vi "BLED1112-Rx Packet parser (RESPONSE-GAP).vi"(5 "message package":u8[](array[numeric])=[0, 3, 6, 3, 0, 0, 0] format="%02x") -> (0 "message out":u8[](array[numeric])=[0, 3, 6, 3, 0, 0, 0] format="%02x", 1 "Packet OK":bool, 2 "Data Structure":T1={"Message Type (Response)"=0, "Payload length"=3, "Message class"=6, "Message ID"=3, "result"=0, "connection_handle"=0} {"Message class" format="%02x"; "connection_handle" format="%02x"; "result" format="%04x"; "Message ID" format="%02x"; "Message Type (Response)" format="%02x" items=["Command / Response"=0, "Event"=128]})   [LabVIEW 2015]
uses:
  Control-BLED Rx (RESPONSE-GAP).ctl
  Lib_Bled112 toolkit/type_def/message_type.ctl
panel:
  # "Rx Packet parser (RESPONSE GAP)"
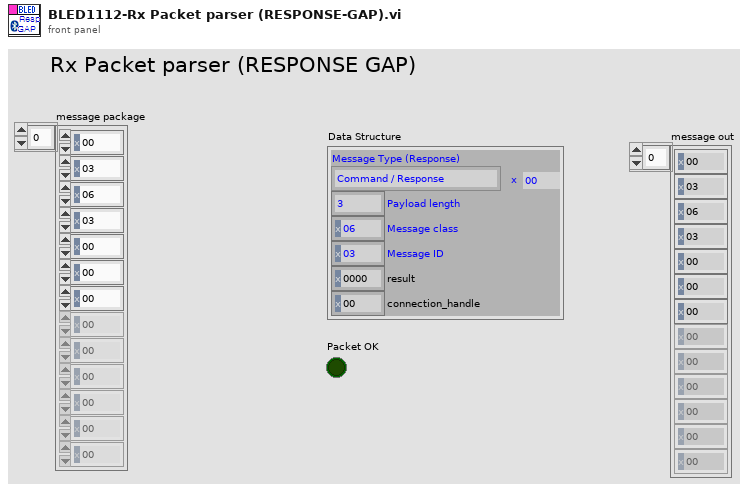
[diagram p1: front panel]
types:
  T1 = typedef "Control-BLED Rx (RESPONSE-GAP).ctl" = cluster{"Message Type (Response)":T2, "Payload length":u8, "Message class":u8, "Message ID":u8, "result":u16, "connection_handle":u8}
  T2 = typedef "message_type.ctl" = u8
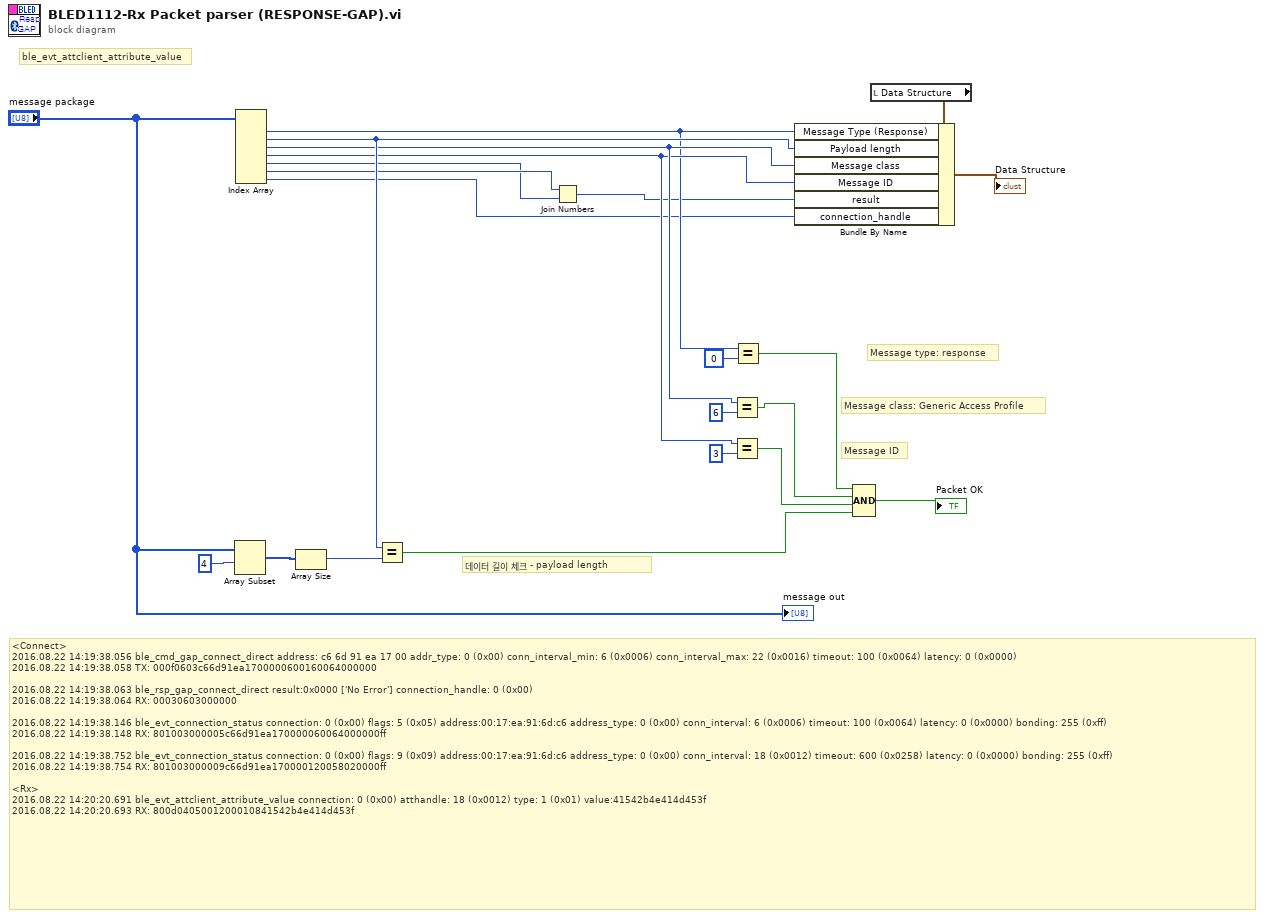
[diagram p0: block diagram]
diagram:
  # "Message type: response"
  # "Message ID"
  # "Message class: Generic Access Profile"
  # "데이터 길이 체크 - payload length"
  # "ble_evt_attclient_attribute_value"
  # "<Connect>\n2016.08.22 14:19:38.056 ble_cmd_gap_connect_direct address: c6 6d 91 ea 17 00 addr_type: 0 (0x00) conn_interval_min: 6 (0x0006) conn_interval_max: 22 (0x0016) timeout: 100 (0x0064) latency: 0 (0x0000)\n2016.08.22 14:19:38.058 TX: 000f0603c66d91ea1700000600160064000000\n\n2016.08.22 14:19:38.063 ble_rsp_gap_connect_direct result:0x0000 ['No Error'] connection_handle: 0 (0x00)\n2016.08.22 14:19:38.064 RX: 00030603000000\n\n2016.08.22 14:19:38.146 ble_evt_connection_status connection: 0 (0x00) flags: 5 (0x05) address:00:17:ea:91:6d:c6 address_type: 0 (0x00) conn_interval: 6 (0x0006) timeout: 100 (0x0064) latency: 0 (0x0000) bonding: 255 (0xff)\n2016.08.22 14:19:38.148 RX: 801003000005c66d91ea170000060064000000ff\n\n2016.08.22 14:19:38.752 ble_evt_connection_status connection: 0 (0x00) flags: 9 (0x09) address:00:17:ea:91:6d:c6 address_type: 0 (0x00) conn_interval: 18 (0x0012) timeout: 600 (0x0258) latency: 0 (0x0000) bonding: 255 (0xff)\n2016.08.22 14:19:38.754 RX: 801003000009c66d91ea170000120058020000ff\n\n<Rx>\n2016.08.22 14:20:20.691 ble_evt_attclient_attribute_value connection: 0 (0x00) atthandle: 18 (0x0012) type: 1 (0x01) value:41542b4e414d453f\n2016.08.22 14:20:20.693 RX: 800d0405001200010841542b4e414d453f"
  n1 = Array Subset(array="message package", index=4 ("인덱스")) -> (w18:u8[])  [unwired: 1 in]
  n2 = Index Array(array="message package") -> (element #1=w5:u8, element #2=w20:u8, element #3=w9:u8, element #4=w8:u8, element #5=w3:u8, element #6=w4:u8, element #7=w1:u8)  [unwired: 7 in]
  n3 = Array Size(array=w18) -> (size(s)=w17:i32)
  n4 = Equal?(x=w20, y=w17) -> (x = y?=w10:bool)
  n5 = Join Numbers(hi=w4, lo=w3) -> ((hi.lo)=w2:u16)
  n6 = Equal?(x=w9, y=6 ("인덱스")) -> (x = y?=w12:bool)
  n7 = Equal?(x=w8, y=3 ("인덱스")) -> (x = y?=w13:bool)
  n8 = Equal?(x=w5, y=0 ("인덱스")) -> (x = y?=w6:bool)
  n9 = Compound Arithmetic op=AND ("복합 연산")(w6, w12, w13, w10) -> (→"Packet OK":bool)
  n10 = local read "Data Structure"() -> (w22:T1)
  n11 = Bundle By Name(cluster=w22, "Message Type (Response)"=w5, "Payload length"=w20, "Message class"=w9, "Message ID"=w8, "result"=w2, "connection_handle"=w1) -> (→"Data Structure":T1)
  "message out" <- "message package"
